vi "Split Text Into Words.vi"(11 "VI Name":string) -> (3 "Array":string[](array[string]))   [LabVIEW 2021, in "Text-Based VI Icon.lvlib"]
uses:
  Text-Based VI Icon.lvlib
  <vilib>/regexp/Match Regular Expression.xnode
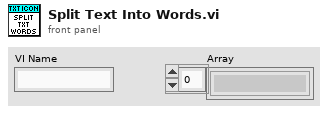
[diagram p1: front panel]
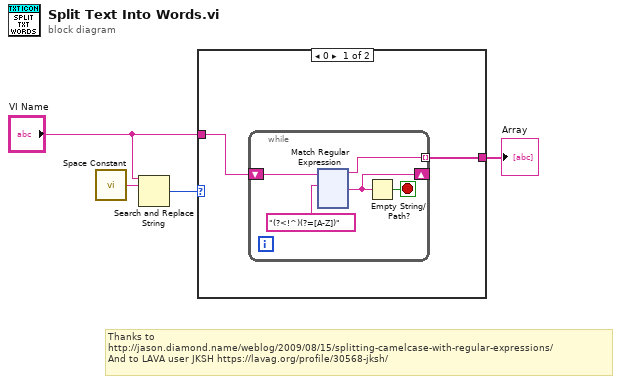
[diagram p0: block diagram]
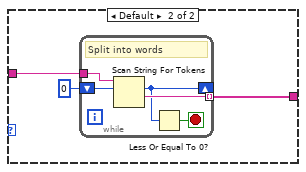
[diagram p2: hidden frame]
diagram:
  # "Thanks to\nhttp://jason.diamond.name/weblog/2009/08/15/splitting-camelcase-with-regular-expressions/\nAnd to LAVA user JKSH https://lavag.org/profile/30568-jksh/"
  n1 = call <vilib>:"Space Constant.vi"() -> ("String"=w3:string)
  n2 = Search and Replace String(input string="VI Name", search string=w3) -> (number of replacements=w2:i32)  [unwired: 6 in, 3 out]
  n3 = case shown="0" w2 {
    tunnel: [w5 w131] -> w4
    tunnel: "VI Name" -> [w6 w129]
    frame 0 {
      n4 = while {
        shift-right: [w8] -> _
        shift-left: w6 -> [w9]
        tunnel: [w7] -> w5 mode=indexing
        stop <- w11 stop-if-true
        n5 = xnode "Match Regular Expression"("input string"=w9, "regular expression"="(?<!^)(?=[A-Z])") -> ("before match"=w7:string, "after match"=w8:string)  [unwired: 4 in, 3 out]
        n6 = Empty String/Path?(string/path=w8) -> (empty?=w11:bool)
      }
    }
    frame Default {
      n7 = while {
        tunnel: w129 -> [w136]
        shift-right: [w133] -> _
        shift-left: 0 ("offset past token") -> [w135]
        tunnel: [w134] -> w131 mode=indexing
        stop <- w132 stop-if-true
        # "Split into words"
        n8 = Scan String For Tokens(8:w135, 9:w136) -> (1:w134:string, 2:w133:i32)  [unwired: 4 in, 2 out]
        n9 = Less Or Equal To 0?(x=w133) -> (x <= 0?=w132:bool)
      }
    }
  }
  "Array" <- w4
